vi "Read Requirements Path.vi"(11 "Project in":refnum<class "RequirementMap.lvclass">) -> (2 "URI":string, 3 "Project out":refnum<class "RequirementMap.lvclass">)   [LabVIEW 2021, in "Bananas.lvlib" / "RequirementMap.lvclass"]
uses:
  RequirementMap.lvclass
  RequirementMap.lvclass/RequirementMap.ctl
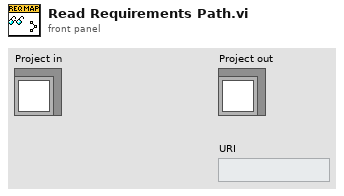
[diagram p1: front panel]
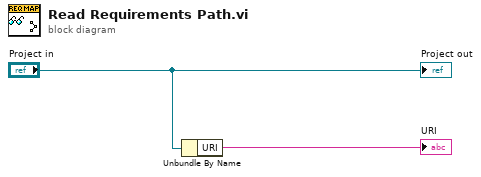
[diagram p0: block diagram]
diagram:
  n1 = Unbundle By Name("Project in") -> ("URI"=→"URI":string)
  "Project out" <- "Project in"
